vi "SubVI de Flip Flop JK.vi"(9 "K":bool, 10 "Q2":bool, 11 "J":bool) -> (3 "Q2*":bool)   [LabVIEW 2018]
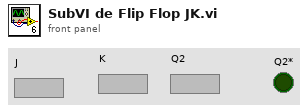
[diagram p1: front panel]
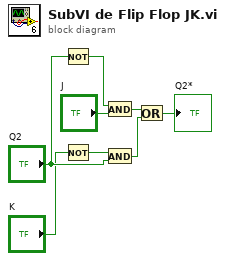
[diagram p0: block diagram]
diagram:
  n1 = Not(x="Q2") -> (.not. x?=w1:bool)
  n2 = Not(x="K") -> (.not. x?=w4:bool)
  n3 = And(x=w1, y="J") -> (x .and. y?=w6:bool)
  n4 = And(x=w4, y="Q2") -> (x .and. y?=w7:bool)
  n5 = Or(x=w6, y=w7) -> (x .or. y?=→"Q2*":bool)
